vi "device_info.vi"(0 "VISA Refnum in":refnum<visa-resource-name>, 1 "error in (no error)":errorcluster) -> (2 "VISA Refnum out":refnum<visa-resource-name>, 3 "concatenated string":string, 4 "error out":errorcluster)   [LabVIEW 2013]
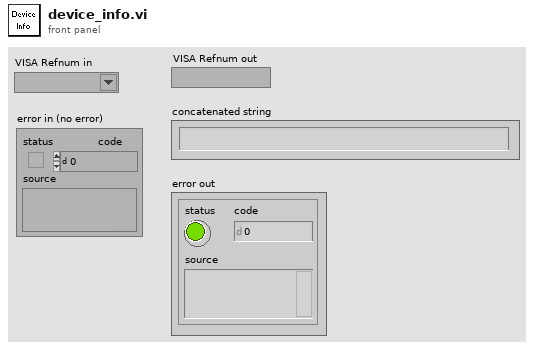
[diagram p1: front panel]
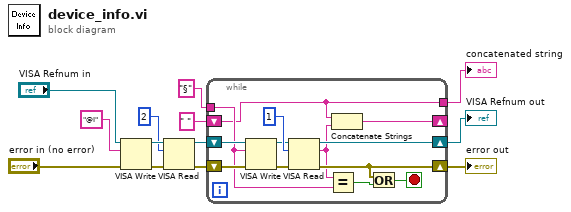
[diagram p0: block diagram]
diagram:
  n1 = VISA Write(VISA resource name="VISA Refnum in", write buffer="@I", error in (no error)="error in (no error)") -> (VISA resource name out=w5:refnum<visa-resource-name>, error out=w4:errorcluster)  [unwired: 1 out]
  n2 = VISA Read(VISA resource name=w5, byte count=u32 2, error in (no error)=w4) -> (VISA resource name out=w3:refnum<visa-resource-name>, error out=w1:errorcluster)  [unwired: 2 out]
  n3 = while {
    tunnel: "§" ("write buffer") -> [w17]
    shift-right: [w23] -> w10
    shift-left: w3 -> [w22]
    shift-right: [w19] -> w11
    shift-left: w1 -> [w21]
    shift-right: [w14] -> _
    shift-left: " " ("string") -> [w15]
    tunnel: [w15] -> w13
    stop <- w20 stop-if-true
    n4 = VISA Write(VISA resource name=w22, write buffer=w17, error in (no error)=w21) -> (VISA resource name out=w25:refnum<visa-resource-name>, error out=w24:errorcluster)  [unwired: 1 out]
    n5 = VISA Read(VISA resource name=w25, byte count=u32 1, error in (no error)=w24) -> (VISA resource name out=w23:refnum<visa-resource-name>, read buffer=w16:string, error out=w19:errorcluster)  [unwired: 1 out]
    n6 = Equal?(x=w16, y=w17) -> (x = y?=w18:bool)
    n7 = Concatenate Strings(w15, w16) -> (w14:string)
    n8 = Or(x=w19, y=w18) -> (x .or. y?=w20:bool)
  }
  "VISA Refnum out" <- w10
  "error out" <- w11
  "concatenated string" <- w13
